vi "sub vi - calibration v1.vi"(11 "Temp Test Cal":dbl) -> ()   [LabVIEW 2013]
uses:
  <vilib>/Platform/TimedLoop/XDataNode/timing_clust.ctl
  <vilib>/Platform/TimedLoop/XDataNode/nitl_modes.ctl
  <vilib>/Platform/TimedLoop/XDataNode/wakeup.ctl
  <vilib>/platform/TimedLoop/XDataNode/XDataNode.xnode
  <vilib>/Platform/TimedLoop/XDataNode/XDNodeRunTimeDep.lvlib
panel:
  out "UPDATE":bool
  in  "stop":bool
  in  "Tab Control":T1(tab)
  out "1-2(TN) Run":dbl
  out "1-2(TL) Run":dbl
  out "1-1(TN) Run":dbl
  out "1-1(TL) Run":dbl
  out "LAB01-1 (GRAPH)":dynamicdata(graph)
  out "LAB01-2 (GRAPH)":dynamicdata(graph)
  in  "LAB01 (CAL)":T2 {"2 (TN) cal" min=0.0 step=0.01 format="%.2f"; "2 (TL) cal" min=0.0 step=0.01 format="%.2f"; "2 (PF) cal" min=0.0 step=0.01 format="%.2f"; "2 (V) cal" min=0.0 step=0.01 format="%.2f"; "2 (A) cal" min=0.0 step=0.01 format="%.2f"; "1 (TN) cal" min=0.0 step=0.01 format="%.2f"; "1 (TL) cal" min=0.0 step=0.01 format="%.2f"; "1 (PF) cal" min=0.0 step=0.01 format="%.2f"; "1 (V) cal" min=0.0 step=0.01 format="%.2f"; "1  (A) cal" min=0.0 step=0.01 format="%.2f"}
  out "LAB01 (SIGNALS)":T3 {"2 (PF)" format="%.2f"; "2 (A)" format="%.1f"; "1 (PF)" format="%.2f"; "1 (A)" format="%.1f"}
  out "2-2(TN) Run":dbl
  out "2-2(TL) Run":dbl
  out "2-1(TN) Run":dbl
  out "2-1(TL) Run":dbl
  out "LAB02 (SIGNALS)":T3 {"2 (PF)" format="%.2f"; "2 (A)" format="%.1f"; "1 (PF)" format="%.2f"; "1 (A)" format="%.1f"}
  in  "LAB02 (CAL)":T4 {"2 (TN) cal" min=0.0 step=0.01 format="%.2f"; "2 (TL) cal" min=0.0 step=0.01 format="%.2f"; "2 (PF) cal" min=0.0 step=0.01 format="%.2f"; "2 (V) cal" min=0.0 step=0.01 format="%.2f"; "2 (A) cal" min=0.0 step=0.01 format="%.2f"; "1 (TN) cal" min=0.0 step=0.01 format="%.2f"; "1 (TL) cal" min=0.0 step=0.01 format="%.2f"; "1 (PF) cal" min=0.0 step=0.01 format="%.2f"; "1 (V) cal" min=0.0 step=0.01 format="%.2f"; "1 (A) cal" min=0.0 step=0.01 format="%.2f"}
  out "LAB02-2 (GRAPH)":dynamicdata(graph)
  out "LAB02-1 (GRAPH)":dynamicdata(graph)
  out "3-2(TN) Run":dbl
  out "3-2(TL) Run":dbl
  out "3-1(TN) Run":dbl
  out "3-1(TL) Run":dbl
  out "LAB03 (SIGNALS)":T3 {"2 (PF)" format="%.2f"; "2 (A)" format="%.1f"; "1 (PF)" format="%.2f"; "1 (A)" format="%.1f"}
  in  "LAB03 (CAL)":T2 {"2 (TN) cal" min=0.0 step=0.01 format="%.2f"; "2 (TL) cal" min=0.0 step=0.01 format="%.2f"; "2 (PF) cal" min=0.0 step=0.01 format="%.2f"; "2 (V) cal" min=0.0 step=0.01 format="%.2f"; "2 (A) cal" min=0.0 step=0.01 format="%.2f"; "1 (TN) cal" min=0.0 step=0.01 format="%.2f"; "1 (TL) cal" min=0.0 step=0.01 format="%.2f"; "1 (PF) cal" min=0.0 step=0.01 format="%.2f"; "1 (V) cal" min=0.0 step=0.01 format="%.2f"; "1  (A) cal" min=0.0 step=0.01 format="%.2f"}
  out "LAB03-2 (GRAPH)":dynamicdata(graph)
  out "LAB03-1 (GRAPH)":dynamicdata(graph)
  out "4-2(TN) Run":dbl
  out "4-2(TL) Run":dbl
  out "4-1(TN) Run":dbl
  out "4-1(TL) Run":dbl
  out "LAB04 (SIGNALS)":T3 {"2 (PF)" format="%.2f"; "2 (A)" format="%.1f"; "1 (PF)" format="%.2f"; "1 (A)" format="%.1f"}
  in  "LAB04 (CAL)":T2 {"2 (TN) cal" min=0.0 step=0.01 format="%.2f"; "2 (TL) cal" min=0.0 step=0.01 format="%.2f"; "2 (PF) cal" min=0.0 step=0.01 format="%.2f"; "2 (V) cal" min=0.0 step=0.01 format="%.2f"; "2 (A) cal" min=0.0 step=0.01 format="%.2f"; "1 (TN) cal" min=0.0 step=0.01 format="%.2f"; "1 (TL) cal" min=0.0 step=0.01 format="%.2f"; "1 (PF) cal" min=0.0 step=0.01 format="%.2f"; "1 (V) cal" min=0.0 step=0.01 format="%.2f"; "1  (A) cal" min=0.0 step=0.01 format="%.2f"}
  out "LAB04-2 (GRAPH)":dynamicdata(graph)
  out "LAB04-1 (GRAPH)":dynamicdata(graph)
  out "5-2(TN) Run":dbl
  out "5-2(TL) Run":dbl
  out "5-1(TN) Run":dbl
  out "5-1(TL) Run":dbl
  out "LAB05 (SIGNALS)":T3 {"2 (PF)" format="%.2f"; "2 (A)" format="%.1f"; "1 (PF)" format="%.2f"; "1 (A)" format="%.1f"}
  in  "LAB05 (CAL)":T2 {"2 (TN) cal" min=0.0 step=0.01 format="%.2f"; "2 (TL) cal" min=0.0 step=0.01 format="%.2f"; "2 (PF) cal" min=0.0 step=0.01 format="%.2f"; "2 (V) cal" min=0.0 step=0.01 format="%.2f"; "2 (A) cal" min=0.0 step=0.01 format="%.2f"; "1 (TN) cal" min=0.0 step=0.01 format="%.2f"; "1 (TL) cal" min=0.0 step=0.01 format="%.2f"; "1 (PF) cal" min=0.0 step=0.01 format="%.2f"; "1 (V) cal" min=0.0 step=0.01 format="%.2f"; "1  (A) cal" min=0.0 step=0.01 format="%.2f"}
  out "LAB05-2 (GRAPH)":dynamicdata(graph)
  out "LAB05-1 (GRAPH)":dynamicdata(graph)
  in  "TEMP REF cal":dbl
  out "AMBIENT TEMP REF":dbl format="%.1f"
  out "Temperature data error":bool
  out "file error out":errorcluster
  out "Analog Loop Time":dbl
  out "analog read ERROR":errorcluster[](array[cluster])
  # "This value is only applied during\ntesting to adjust for insulatred probe\nprofile during current flow temp rise.\nIf any change is made here, make sure\nvalue is changed to same value on\nADM tab."
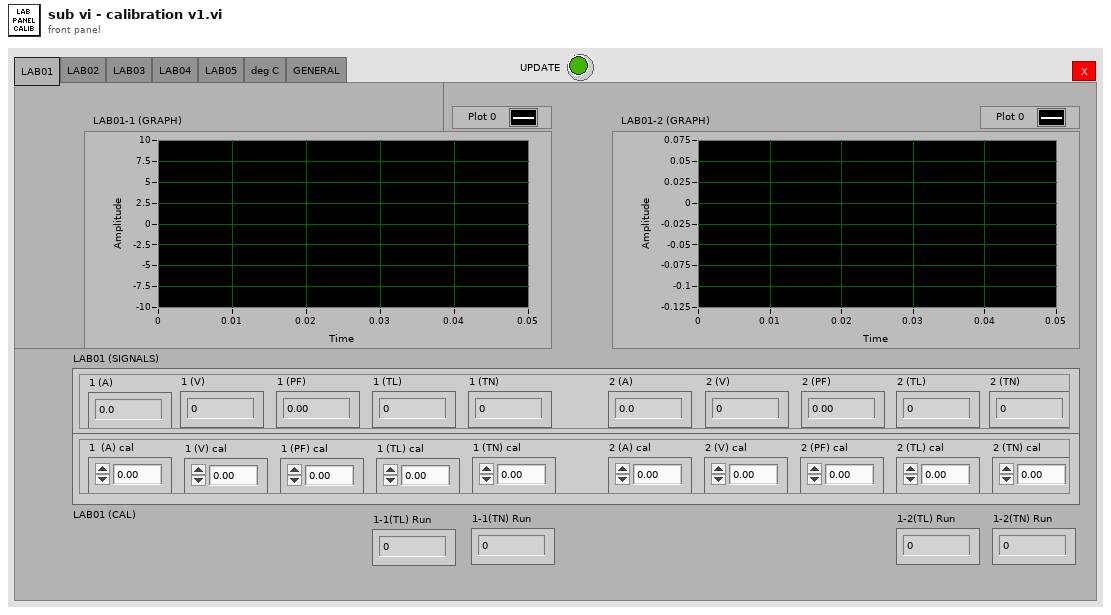
[diagram p1: front panel]
types:
  T1 = enum32{"LAB01", "LAB02", "LAB03", "LAB04", "LAB05", "deg C", "GENERAL"}
  T2 = cluster{"1  (A) cal":dbl, "1 (V) cal":dbl, "1 (PF) cal":dbl, "1 (TL) cal":dbl, "1 (TN) cal":dbl, "2 (A) cal":dbl, "2 (V) cal":dbl, "2 (PF) cal":dbl, "2 (TL) cal":dbl, "2 (TN) cal":dbl}
  T3 = cluster{"1 (TL)":dbl, "1 (TN)":dbl, "2 (TL)":dbl, "2 (TN)":dbl, "1 (A)":dbl, "1 (V)":dbl, "1 (PF)":dbl, "2 (A)":dbl, "2 (V)":dbl, "2 (PF)":dbl}
  T4 = cluster{"1 (A) cal":dbl, "1 (V) cal":dbl, "1 (PF) cal":dbl, "1 (TL) cal":dbl, "1 (TN) cal":dbl, "2 (A) cal":dbl, "2 (V) cal":dbl, "2 (PF) cal":dbl, "2 (TL) cal":dbl, "2 (TN) cal":dbl}
  T5 = enum16{"open", "replace", "create", "open or create", "replace or create", "replace or create with confirmation"}
  T6 = typedef "XDNodeRunTimeDep.lvlib/timing_clust.ctl" = cluster{"Expected End [f-1]":u64, "Actual End [f-1]":u64, "Finished Late? [f-1]":bool, "Expected End [i-1]":u64, "Actual End [i-1]":u64, "Finished Late? [i-1]":bool, "Expected Start [i]":u64, "Actual Start [i]":u64, "Expected Start [f]":u64, "Actual Start [f]":u64, "Source Name":string, "Structure Name":string, "Period":i64, "Deadline":i64, "Offset":i64, "Start":i64, "Priority":i32, "Timeout":i32, "Mode":T7, "Wakeup Reason":T8, "Error":errorcluster, "Source Type":string, "Secondary Source Type":string, "Global End Time":u64, "Global Start Time":u64, "Frame Duration":u64, "Iteration Duration":u64, "Assigned CPU":i32, "I/O Scan Engine Mode":u32}
  T7 = typedef "XDNodeRunTimeDep.lvlib/nitl_modes.ctl" = enum32{"No Change", "Process missed periods, maintain original phase", "Discard missed periods, maintain original phase", "Process missed periods, ignore original phase", "Discard missed periods, ignore original phase"}
  T8 = typedef "XDNodeRunTimeDep.lvlib/wakeup.ctl" = enum32{"Normal", "Aborted", "Asynchronous wakeup", "Timing source error", "Timed loop error", "Timeout"}
  T9 = cluster{"LAB01-1 (A)":dbl, "LAB01-1 (V)":dbl, "LAB01-1 (PF)":dbl, "LAB01-2 (A)":dbl, "LAB01-2 (V)":dbl, "LAB01-2 (PF)":dbl}
  T10 = cluster{"LAB02-1 (A)":dbl, "LAB02-1 (V)":dbl, "LAB02-1 (PF)":dbl, "LAB02-2 (A)":dbl, "LAB02-2 (V)":dbl, "LAB02-2 (PF)":dbl}
  T11 = cluster{"LAB03-1 (A)":dbl, "LAB03-1 (V)":dbl, "LAB03-1 (PF)":dbl, "LAB03-2 (A)":dbl, "LAB03-2 (V)":dbl, "LAB03-2 (PF)":dbl}
  T12 = cluster{"LAB04-1 (A)":dbl, "LAB04-1 (V)":dbl, "LAB04-1 (PF)":dbl, "LAB04-2 (A)":dbl, "LAB04-2 (V)":dbl, "LAB04-2 (PF)":dbl}
  T13 = cluster{"LAB05-1 (A)":dbl, "LAB05-1 (V)":dbl, "LAB05-1 (PF)":dbl, "LAB05-2 (A)":dbl, "LAB05-2 (V)":dbl, "LAB05-2 (PF)":dbl}
  T14 = cluster{"T1":dbl, "T2":dbl, "T3":dbl, "T4":dbl, "ID":dbl, "ER":dbl}
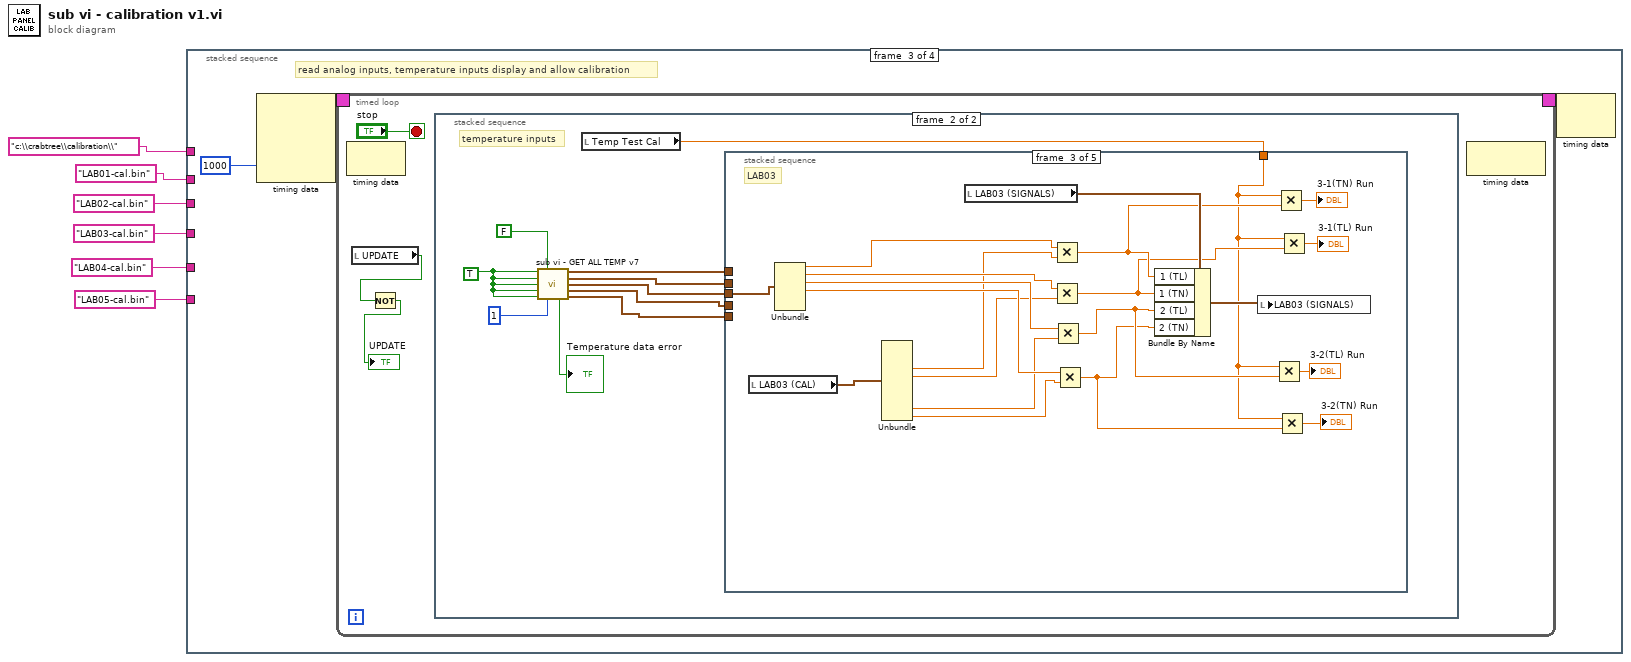
[diagram p0: block diagram]
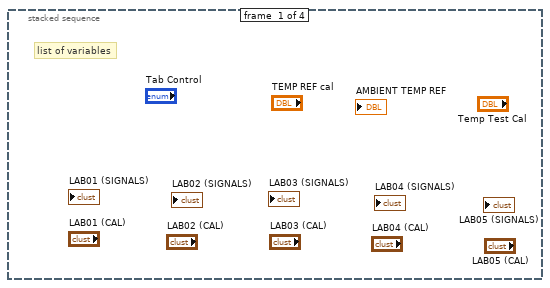
[diagram p2: hidden frame]
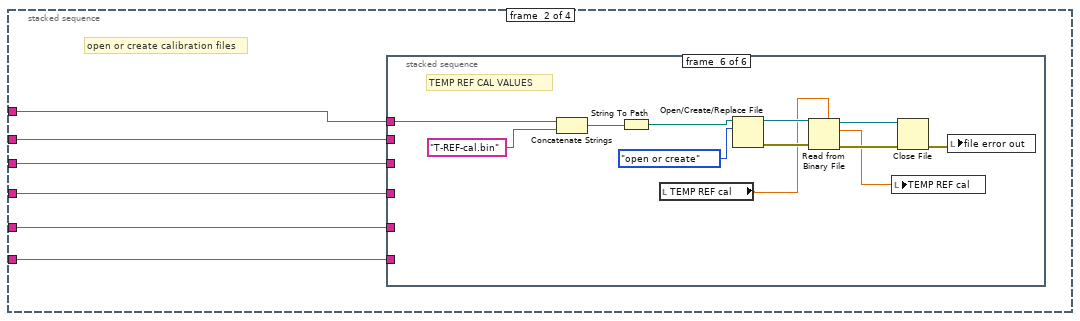
[diagram p3: hidden frame]
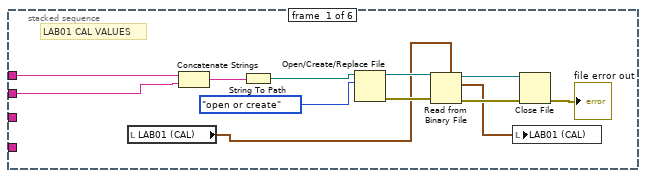
[diagram p4: hidden frame]
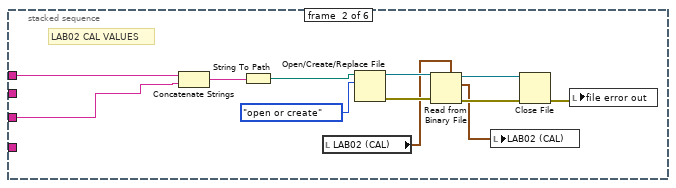
[diagram p5: hidden frame]
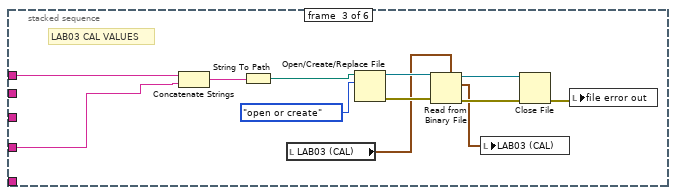
[diagram p6: hidden frame]
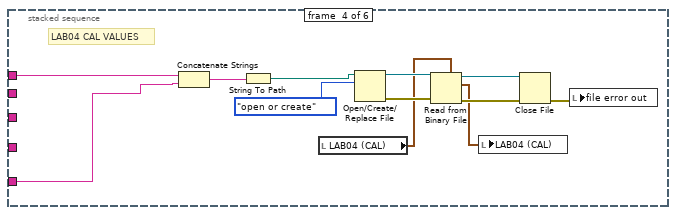
[diagram p7: hidden frame]
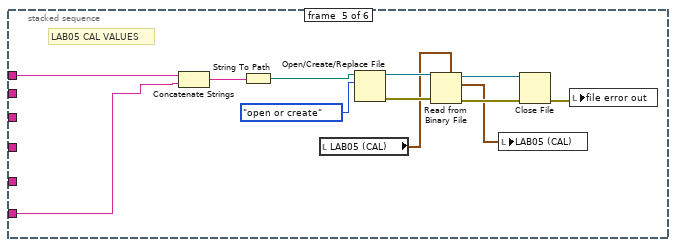
[diagram p8: hidden frame]
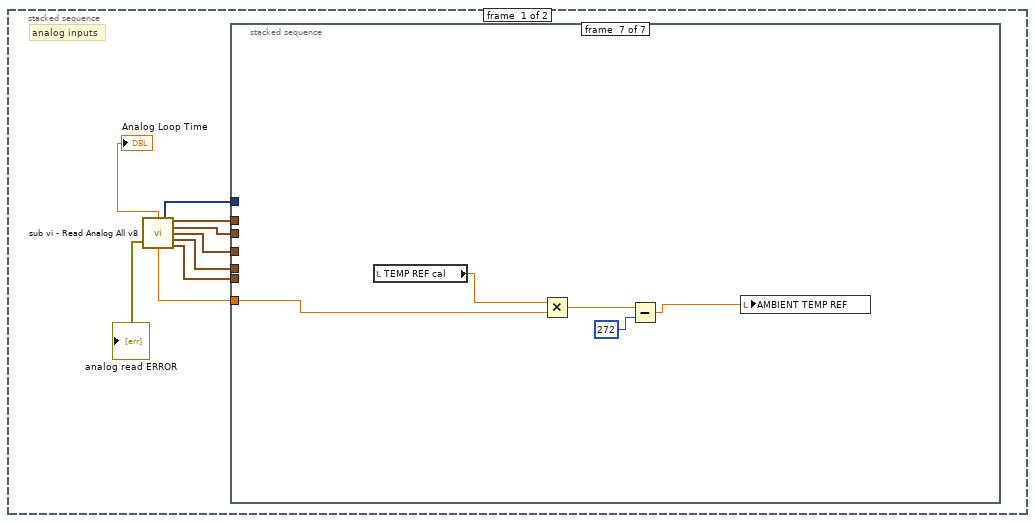
[diagram p9: hidden frame]
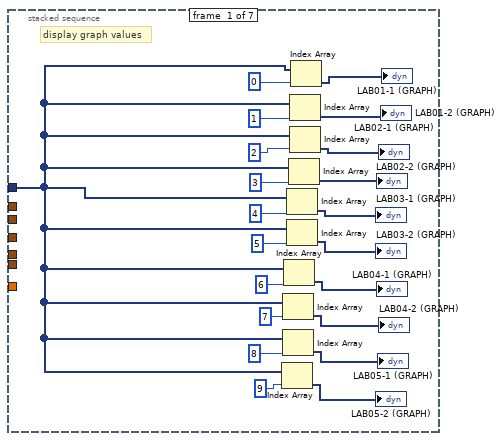
[diagram p10: hidden frame]
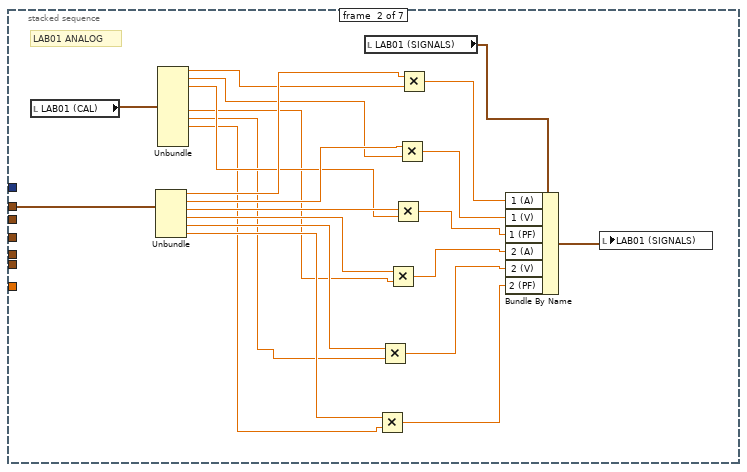
[diagram p11: hidden frame]
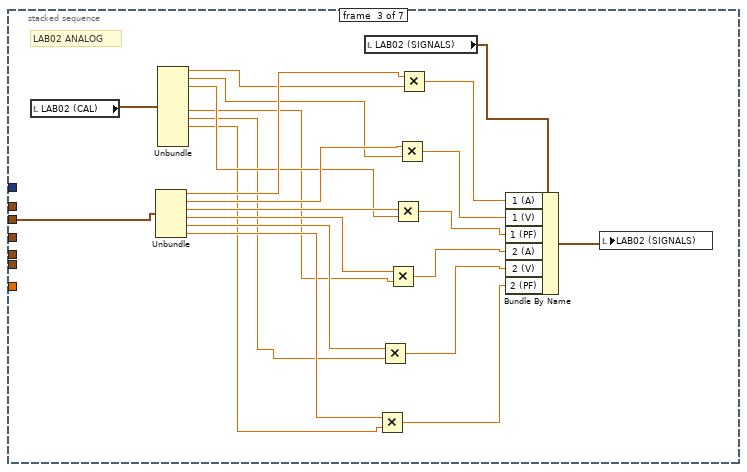
[diagram p12: hidden frame]
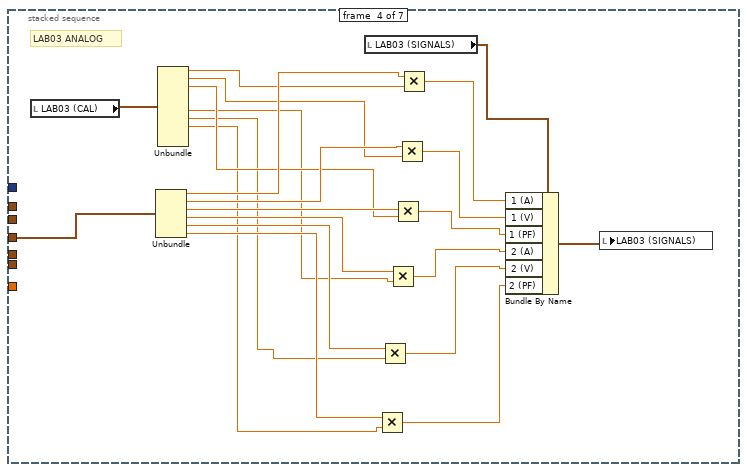
[diagram p13: hidden frame]
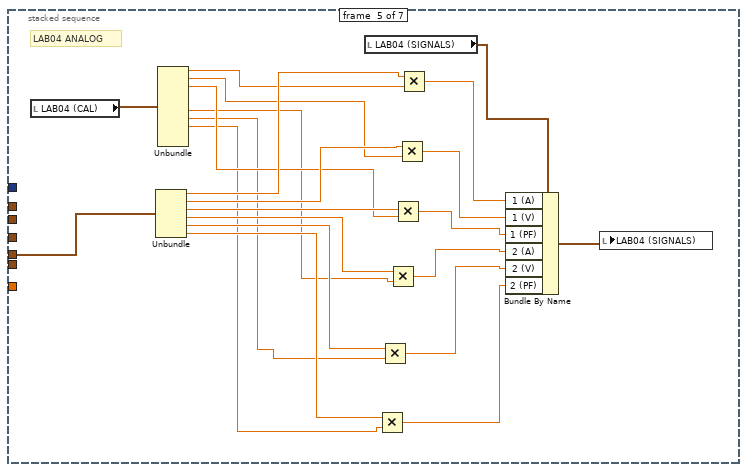
[diagram p14: hidden frame]
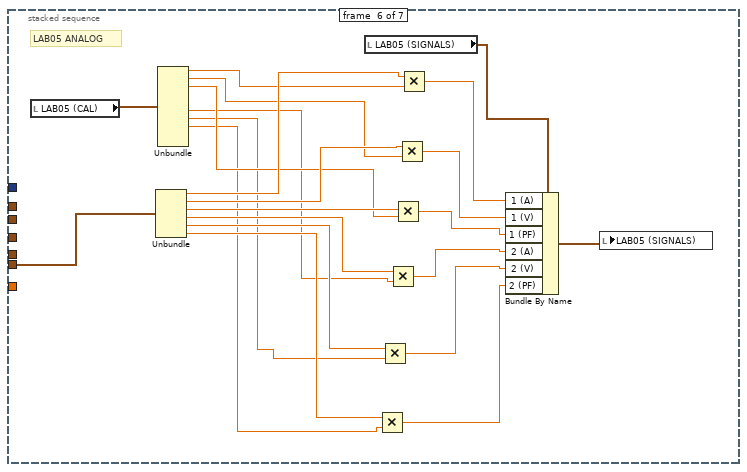
[diagram p15: hidden frame]
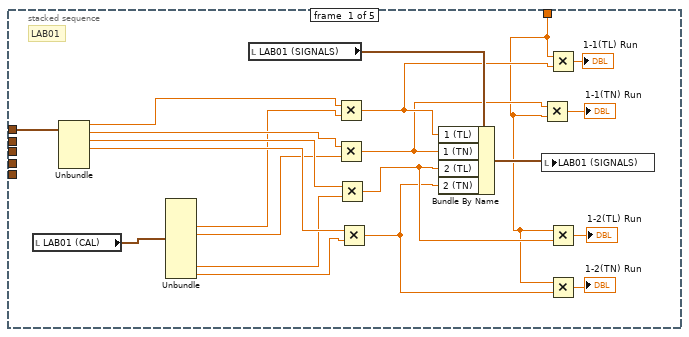
[diagram p16: hidden frame]
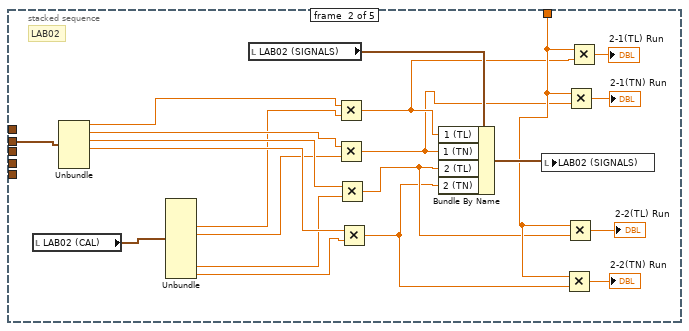
[diagram p17: hidden frame]
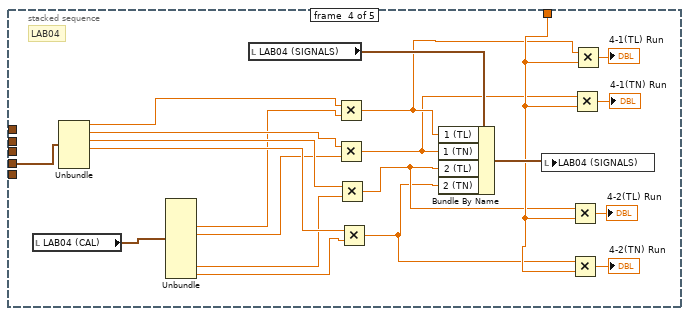
[diagram p18: hidden frame]
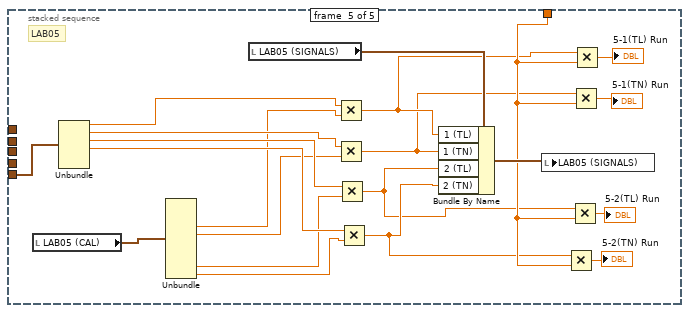
[diagram p19: hidden frame]
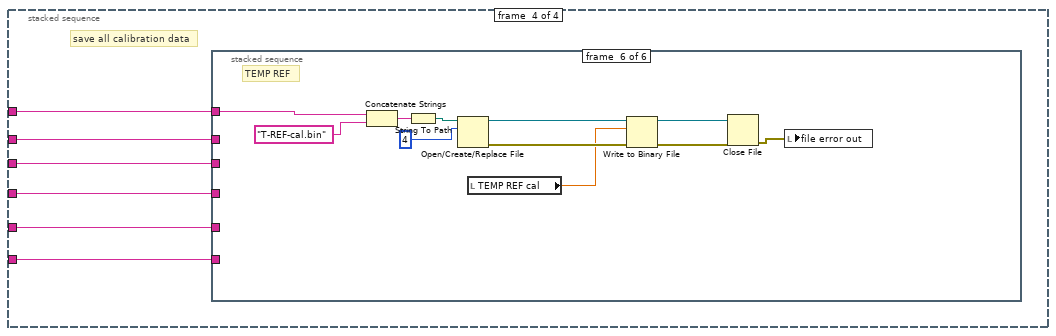
[diagram p20: hidden frame]
diagram:
  n1 = stacked-sequence {
    tunnel: "c:\\crabtree\\calibration\\" -> [_ w12 _ w362]
    tunnel: "LAB01-cal.bin" -> [_ w11 _ w361]
    tunnel: "LAB02-cal.bin" -> [_ w10 _ w360]
    tunnel: "LAB03-cal.bin" -> [_ w9 _ w359]
    tunnel: "LAB04-cal.bin" -> [_ w8 _ w358]
    tunnel: "LAB05-cal.bin" -> [_ w7 _ w357]
    frame #0 {
      # "list of variables"
    }
    frame #1 {
      # "open or create calibration files"
      n2 = stacked-sequence {
        tunnel: w12 -> [w24 w36 w48 w60 w72 w84]
        tunnel: w11 -> [w15 _ _ _ _ _]
        tunnel: w10 -> [_ w27 _ _ _ _]
        tunnel: w9 -> [_ _ w39 _ _ _]
        tunnel: w8 -> [_ _ _ w52 _ _]
        tunnel: w7 -> [_ _ _ _ w63 _]
        frame #0 {
          # "LAB01 CAL VALUES"
          n3 = local read "LAB01 (CAL)"() -> (w14:T2)
          n4 = Concatenate Strings(w24, w15) -> (w23:string)
          n5 = String To Path(string=w23) -> (path=w22:path)
          n6 = Open/Create/Replace File(file path (use dialog)=w22, operation (0:open)=T5."open or create") -> (refnum out=w21:refnum<file>, error out=w20:errorcluster)  [unwired: 4 in, 1 out]
          n7 = Read from Binary File(5:w14, 8:w20, 11:w21) -> (0:w18:errorcluster, 2:w13:T2, 3:w19:refnum<file>)  [unwired: 3 in, 1 out]
          n8 = local write "LAB01 (CAL)"(w13) -> ()
          n9 = Close File(refnum=w19, error in=w18) -> (error out=→"file error out":errorcluster)  [unwired: 1 out]
        }
        frame #1 {
          # "LAB02 CAL VALUES"
          n10 = Concatenate Strings(w36, w27) -> (w35:string)
          n11 = String To Path(string=w35) -> (path=w34:path)
          n12 = local read "LAB02 (CAL)"() -> (w26:T4)
          n13 = Open/Create/Replace File(file path (use dialog)=w34, operation (0:open)=T5."open or create") -> (refnum out=w33:refnum<file>, error out=w32:errorcluster)  [unwired: 4 in, 1 out]
          n14 = Read from Binary File(5:w26, 8:w32, 11:w33) -> (0:w30:errorcluster, 2:w25:T4, 3:w31:refnum<file>)  [unwired: 3 in, 1 out]
          n15 = local write "LAB02 (CAL)"(w25) -> ()
          n16 = Close File(refnum=w31, error in=w30) -> (error out=w28:errorcluster)  [unwired: 1 out]
          n17 = local write "file error out"(w28) -> ()
        }
        frame #2 {
          # "LAB03 CAL VALUES"
          n18 = Concatenate Strings(w48, w39) -> (w47:string)
          n19 = String To Path(string=w47) -> (path=w46:path)
          n20 = local read "LAB03 (CAL)"() -> (w38:T2)
          n21 = Open/Create/Replace File(file path (use dialog)=w46, operation (0:open)=T5."open or create") -> (refnum out=w45:refnum<file>, error out=w44:errorcluster)  [unwired: 4 in, 1 out]
          n22 = Read from Binary File(5:w38, 8:w44, 11:w45) -> (0:w42:errorcluster, 2:w37:T2, 3:w43:refnum<file>)  [unwired: 3 in, 1 out]
          n23 = local write "LAB03 (CAL)"(w37) -> ()
          n24 = Close File(refnum=w43, error in=w42) -> (error out=w40:errorcluster)  [unwired: 1 out]
          n25 = local write "file error out"(w40) -> ()
        }
        frame #3 {
          # "LAB04 CAL VALUES"
          n26 = Concatenate Strings(w60, w52) -> (w59:string)
          n27 = String To Path(string=w59) -> (path=w58:path)
          n28 = local read "LAB04 (CAL)"() -> (w50:T2)
          n29 = Open/Create/Replace File(file path (use dialog)=w58, operation (0:open)=T5."open or create") -> (refnum out=w57:refnum<file>, error out=w56:errorcluster)  [unwired: 4 in, 1 out]
          n30 = Read from Binary File(5:w50, 8:w56, 11:w57) -> (0:w54:errorcluster, 2:w49:T2, 3:w55:refnum<file>)  [unwired: 3 in, 1 out]
          n31 = local write "LAB04 (CAL)"(w49) -> ()
          n32 = Close File(refnum=w55, error in=w54) -> (error out=w53:errorcluster)  [unwired: 1 out]
          n33 = local write "file error out"(w53) -> ()
        }
        frame #4 {
          # "LAB05 CAL VALUES"
          n34 = Concatenate Strings(w72, w63) -> (w71:string)
          n35 = String To Path(string=w71) -> (path=w70:path)
          n36 = local read "LAB05 (CAL)"() -> (w62:T2)
          n37 = Open/Create/Replace File(file path (use dialog)=w70, operation (0:open)=T5."open or create") -> (refnum out=w69:refnum<file>, error out=w68:errorcluster)  [unwired: 4 in, 1 out]
          n38 = Read from Binary File(5:w62, 8:w68, 11:w69) -> (0:w66:errorcluster, 2:w61:T2, 3:w67:refnum<file>)  [unwired: 3 in, 1 out]
          n39 = local write "LAB05 (CAL)"(w61) -> ()
          n40 = Close File(refnum=w67, error in=w66) -> (error out=w64:errorcluster)  [unwired: 1 out]
          n41 = local write "file error out"(w64) -> ()
        }
        frame #5 {
          # "TEMP REF CAL VALUES"
          n42 = Concatenate Strings(w84, "T-REF-cal.bin") -> (w83:string)
          n43 = String To Path(string=w83) -> (path=w82:path)
          n44 = local read "TEMP REF cal"() -> (w74:dbl)
          n45 = Open/Create/Replace File(file path (use dialog)=w82, operation (0:open)=T5."open or create") -> (refnum out=w81:refnum<file>, error out=w80:errorcluster)  [unwired: 4 in, 1 out]
          n46 = Read from Binary File(5:w74, 8:w80, 11:w81) -> (0:w78:errorcluster, 2:w73:dbl, 3:w79:refnum<file>)  [unwired: 3 in, 1 out]
          n47 = local write "TEMP REF cal"(w73) -> ()
          n48 = Close File(refnum=w79, error in=w78) -> (error out=w76:errorcluster)  [unwired: 1 out]
          n49 = local write "file error out"(w76) -> ()
        }
      }
    }
    frame #2 {
      # "read analog inputs, temperature inputs display and allow calibration"
      n50 = node-c288(1000) -> (w87:T6)  [unwired: 3 in]
      n51 = timed-loop {
        timing: w87 -> [_]
        timing-out: [_] -> w86
        stop <- "stop" stop-if-true
        n52 = node-c288() -> ()  [unwired: 1 in, 1 out]
        n53 = local read "UPDATE"() -> (w88:bool)
        n54 = Not(x=w88) -> (.not. x?=→"UPDATE":bool)
        n55 = stacked-sequence {
          frame #0 {
            # "analog inputs"
            n56 = call "sub vi - Read Analog All v8.vi"() -> ("Analog loop time"=→"Analog Loop Time":dbl, "array GRAPH"=w98:dynamicdata[], "LAB01"=w97:T9, "LAB02"=w95:T10, "LAB03"=w96:T11, "LAB04"=w94:T12, "deg C"=w91:dbl, "array ERROR"=→"analog read ERROR":errorcluster[], "LAB05"=w93:T13)  [unwired: 7 in]
            n57 = stacked-sequence {
              tunnel: w98 -> [w119 _ _ _ _ _ _]
              tunnel: w97 -> [_ w141 _ _ _ _ _]
              tunnel: w96 -> [_ _ _ w165 _ _ _]
              tunnel: w95 -> [_ _ w143 _ _ _ _]
              tunnel: w94 -> [_ _ _ _ w187 _ _]
              tunnel: w93 -> [_ _ _ _ _ w209 _]
              tunnel: w91 -> [_ _ _ _ _ _ w234]
              frame #0 {
                # "display graph values"
                n58 = Index Array(array=w119, index=9) -> (element=→"LAB05-2 (GRAPH)":dynamicdata)
                n59 = Index Array(array=w119, index=7) -> (element=→"LAB04-2 (GRAPH)":dynamicdata)
                n60 = Index Array(array=w119, index=8) -> (element=→"LAB05-1 (GRAPH)":dynamicdata)
                n61 = Index Array(array=w119, index=6) -> (element=→"LAB04-1 (GRAPH)":dynamicdata)
                n62 = Index Array(array=w119, index=4) -> (element=→"LAB03-1 (GRAPH)":dynamicdata)
                n63 = Index Array(array=w119, index=5) -> (element=→"LAB03-2 (GRAPH)":dynamicdata)
                n64 = Index Array(array=w119, index=3) -> (element=→"LAB02-2 (GRAPH)":dynamicdata)
                n65 = Index Array(array=w119, index=1) -> (element=→"LAB01-2 (GRAPH)":dynamicdata)
                n66 = Index Array(array=w119, index=2) -> (element=→"LAB02-1 (GRAPH)":dynamicdata)
                n67 = Index Array(array=w119, index=0) -> (element=→"LAB01-1 (GRAPH)":dynamicdata)
              }
              frame #1 {
                # "LAB01 ANALOG"
                n68 = local read "LAB01 (CAL)"() -> (w142:T2)
                n69 = Unbundle(w141) -> ("LAB01-1 (A)"=w140:dbl, "LAB01-1 (V)"=w139:dbl, "LAB01-1 (PF)"=w138:dbl, "LAB01-2 (A)"=w137:dbl, "LAB01-2 (V)"=w136:dbl, "LAB01-2 (PF)"=w135:dbl)
                n70 = Unbundle(w142) -> ("1  (A) cal"=w134:dbl, "1 (V) cal"=w133:dbl, "1 (PF) cal"=w132:dbl, "2 (A) cal"=w131:dbl, "2 (V) cal"=w130:dbl, "2 (PF) cal"=w129:dbl)  [unwired: 4 out]
                n71 = local read "LAB01 (SIGNALS)"() -> (w128:T3)
                n72 = Multiply(x=w135, y=w129) -> (x*y=w122:dbl)
                n73 = Multiply(x=w136, y=w130) -> (x*y=w123:dbl)
                n74 = Multiply(x=w137, y=w131) -> (x*y=w124:dbl)
                n75 = Multiply(x=w138, y=w132) -> (x*y=w125:dbl)
                n76 = Multiply(x=w139, y=w133) -> (x*y=w126:dbl)
                n77 = Multiply(x=w140, y=w134) -> (x*y=w127:dbl)
                n78 = Bundle By Name(cluster=w128, "1 (A)"=w127, "1 (V)"=w126, "1 (PF)"=w125, "2 (A)"=w124, "2 (V)"=w123, "2 (PF)"=w122) -> (w121:T3)
                n79 = local write "LAB01 (SIGNALS)"(w121) -> ()
              }
              frame #2 {
                # "LAB02 ANALOG"
                n80 = local read "LAB02 (CAL)"() -> (w164:T4)
                n81 = Unbundle(w143) -> ("LAB02-1 (A)"=w163:dbl, "LAB02-1 (V)"=w162:dbl, "LAB02-1 (PF)"=w161:dbl, "LAB02-2 (A)"=w160:dbl, "LAB02-2 (V)"=w159:dbl, "LAB02-2 (PF)"=w158:dbl)
                n82 = Unbundle(w164) -> ("1 (A) cal"=w157:dbl, "1 (V) cal"=w156:dbl, "1 (PF) cal"=w155:dbl, "2 (A) cal"=w154:dbl, "2 (V) cal"=w153:dbl, "2 (PF) cal"=w152:dbl)  [unwired: 4 out]
                n83 = local read "LAB02 (SIGNALS)"() -> (w151:T3)
                n84 = Multiply(x=w158, y=w152) -> (x*y=w145:dbl)
                n85 = Multiply(x=w159, y=w153) -> (x*y=w146:dbl)
                n86 = Multiply(x=w160, y=w154) -> (x*y=w147:dbl)
                n87 = Multiply(x=w161, y=w155) -> (x*y=w148:dbl)
                n88 = Multiply(x=w162, y=w156) -> (x*y=w149:dbl)
                n89 = Multiply(x=w163, y=w157) -> (x*y=w150:dbl)
                n90 = Bundle By Name(cluster=w151, "1 (A)"=w150, "1 (V)"=w149, "1 (PF)"=w148, "2 (A)"=w147, "2 (V)"=w146, "2 (PF)"=w145) -> (w144:T3)
                n91 = local write "LAB02 (SIGNALS)"(w144) -> ()
              }
              frame #3 {
                # "LAB03 ANALOG"
                n92 = local read "LAB03 (CAL)"() -> (w186:T2)
                n93 = Unbundle(w165) -> ("LAB03-1 (A)"=w185:dbl, "LAB03-1 (V)"=w184:dbl, "LAB03-1 (PF)"=w183:dbl, "LAB03-2 (A)"=w182:dbl, "LAB03-2 (V)"=w181:dbl, "LAB03-2 (PF)"=w180:dbl)
                n94 = Unbundle(w186) -> ("1  (A) cal"=w179:dbl, "1 (V) cal"=w178:dbl, "1 (PF) cal"=w177:dbl, "2 (A) cal"=w176:dbl, "2 (V) cal"=w175:dbl, "2 (PF) cal"=w174:dbl)  [unwired: 4 out]
                n95 = local read "LAB03 (SIGNALS)"() -> (w173:T3)
                n96 = Multiply(x=w180, y=w174) -> (x*y=w167:dbl)
                n97 = Multiply(x=w181, y=w175) -> (x*y=w168:dbl)
                n98 = Multiply(x=w182, y=w176) -> (x*y=w169:dbl)
                n99 = Multiply(x=w183, y=w177) -> (x*y=w170:dbl)
                n100 = Multiply(x=w184, y=w178) -> (x*y=w171:dbl)
                n101 = Multiply(x=w185, y=w179) -> (x*y=w172:dbl)
                n102 = Bundle By Name(cluster=w173, "1 (A)"=w172, "1 (V)"=w171, "1 (PF)"=w170, "2 (A)"=w169, "2 (V)"=w168, "2 (PF)"=w167) -> (w166:T3)
                n103 = local write "LAB03 (SIGNALS)"(w166) -> ()
              }
              frame #4 {
                # "LAB04 ANALOG"
                n104 = local read "LAB04 (CAL)"() -> (w208:T2)
                n105 = Unbundle(w187) -> ("LAB04-1 (A)"=w207:dbl, "LAB04-1 (V)"=w206:dbl, "LAB04-1 (PF)"=w205:dbl, "LAB04-2 (A)"=w204:dbl, "LAB04-2 (V)"=w203:dbl, "LAB04-2 (PF)"=w202:dbl)
                n106 = Unbundle(w208) -> ("1  (A) cal"=w201:dbl, "1 (V) cal"=w200:dbl, "1 (PF) cal"=w199:dbl, "2 (A) cal"=w198:dbl, "2 (V) cal"=w197:dbl, "2 (PF) cal"=w196:dbl)  [unwired: 4 out]
                n107 = local read "LAB04 (SIGNALS)"() -> (w195:T3)
                n108 = Multiply(x=w202, y=w196) -> (x*y=w189:dbl)
                n109 = Multiply(x=w203, y=w197) -> (x*y=w190:dbl)
                n110 = Multiply(x=w204, y=w198) -> (x*y=w191:dbl)
                n111 = Multiply(x=w205, y=w199) -> (x*y=w192:dbl)
                n112 = Multiply(x=w206, y=w200) -> (x*y=w193:dbl)
                n113 = Multiply(x=w207, y=w201) -> (x*y=w194:dbl)
                n114 = Bundle By Name(cluster=w195, "1 (A)"=w194, "1 (V)"=w193, "1 (PF)"=w192, "2 (A)"=w191, "2 (V)"=w190, "2 (PF)"=w189) -> (w188:T3)
                n115 = local write "LAB04 (SIGNALS)"(w188) -> ()
              }
              frame #5 {
                # "LAB05 ANALOG"
                n116 = local read "LAB05 (CAL)"() -> (w230:T2)
                n117 = Unbundle(w209) -> ("LAB05-1 (A)"=w229:dbl, "LAB05-1 (V)"=w228:dbl, "LAB05-1 (PF)"=w227:dbl, "LAB05-2 (A)"=w226:dbl, "LAB05-2 (V)"=w225:dbl, "LAB05-2 (PF)"=w224:dbl)
                n118 = Unbundle(w230) -> ("1  (A) cal"=w223:dbl, "1 (V) cal"=w222:dbl, "1 (PF) cal"=w221:dbl, "2 (A) cal"=w220:dbl, "2 (V) cal"=w219:dbl, "2 (PF) cal"=w218:dbl)  [unwired: 4 out]
                n119 = local read "LAB05 (SIGNALS)"() -> (w217:T3)
                n120 = Multiply(x=w224, y=w218) -> (x*y=w211:dbl)
                n121 = Multiply(x=w225, y=w219) -> (x*y=w212:dbl)
                n122 = Multiply(x=w226, y=w220) -> (x*y=w213:dbl)
                n123 = Multiply(x=w227, y=w221) -> (x*y=w214:dbl)
                n124 = Multiply(x=w228, y=w222) -> (x*y=w215:dbl)
                n125 = Multiply(x=w229, y=w223) -> (x*y=w216:dbl)
                n126 = Bundle By Name(cluster=w217, "1 (A)"=w216, "1 (V)"=w215, "1 (PF)"=w214, "2 (A)"=w213, "2 (V)"=w212, "2 (PF)"=w211) -> (w210:T3)
                n127 = local write "LAB05 (SIGNALS)"(w210) -> ()
              }
              frame #6 {
                n128 = local read "TEMP REF cal"() -> (w235:dbl)
                n129 = Multiply(x=w235, y=w234) -> (x*y=w233:dbl)
                n130 = Subtract(x=w233, y=272) -> (x-y=w231:dbl)
                n131 = local write "AMBIENT TEMP REF"(w231) -> ()
              }
            }
          }
          frame #1 {
            w245 = TRUE
            # "temperature inputs"
            n132 = call "sub vi - GET ALL TEMP v7.vi"("LA01-EN"=w245, "simulate"=FALSE, "LA02-EN"=w245, "LA03-EN"=w245, "LA04-EN"=w245, "LA05-EN"=w245, "Gen Cal Value"=1) -> ("LA01 TEMP"=w243:T14, "LA02 TEMP"=w241:T14, "LA03 TEMP"=w240:T14, "LA04 TEMP"=w239:T14, "error"=→"Temperature data error":bool, "LA05 TEMP"=w238:T14)  [unwired: 1 in, 2 out]
            n133 = local read "Temp Test Cal"() -> (w236:dbl)
            n134 = stacked-sequence {
              tunnel: w243 -> [w265 _ _ _ _]
              tunnel: w241 -> [_ w276 _ _ _]
              tunnel: w240 -> [_ _ w297 _ _]
              tunnel: w239 -> [_ _ _ w318 _]
              tunnel: w238 -> [_ _ _ _ w339]
              tunnel: w236 -> [w246 w271 w289 w313 w334]
              frame #0 {
                # "LAB01"
                n135 = local read "LAB01 (CAL)"() -> (w266:T2)
                n136 = Unbundle(w265) -> ("T1"=w264:dbl, "T2"=w263:dbl, "T3"=w262:dbl, "T4"=w261:dbl)  [unwired: 2 out]
                n137 = Unbundle(w266) -> ("1 (TL) cal"=w260:dbl, "1 (TN) cal"=w259:dbl, "2 (TL) cal"=w258:dbl, "2 (TN) cal"=w257:dbl)  [unwired: 6 out]
                n138 = local read "LAB01 (SIGNALS)"() -> (w256:T3)
                n139 = Multiply(x=w264, y=w260) -> (x*y=w253:dbl)
                n140 = Multiply(x=w263, y=w259) -> (x*y=w251:dbl)
                n141 = Multiply(x=w262, y=w258) -> (x*y=w248:dbl)
                n142 = Multiply(x=w261, y=w257) -> (x*y=w247:dbl)
                n143 = Bundle By Name(cluster=w256, "1 (TL)"=w253, "1 (TN)"=w251, "2 (TL)"=w248, "2 (TN)"=w247) -> (w255:T3)
                n144 = Multiply(x=w251, y=w246) -> (x*y=→"1-1(TN) Run":dbl)
                n145 = local write "LAB01 (SIGNALS)"(w255) -> ()
                n146 = Multiply(x=w246, y=w253) -> (x*y=→"1-1(TL) Run":dbl)
                n147 = Multiply(x=w246, y=w248) -> (x*y=→"1-2(TL) Run":dbl)
                n148 = Multiply(x=w246, y=w247) -> (x*y=→"1-2(TN) Run":dbl)
              }
              frame #1 {
                # "LAB02"
                n149 = local read "LAB02 (CAL)"() -> (w287:T4)
                n150 = Unbundle(w276) -> ("T1"=w286:dbl, "T2"=w285:dbl, "T3"=w284:dbl, "T4"=w283:dbl)  [unwired: 2 out]
                n151 = Unbundle(w287) -> ("1 (TL) cal"=w282:dbl, "1 (TN) cal"=w281:dbl, "2 (TL) cal"=w280:dbl, "2 (TN) cal"=w279:dbl)  [unwired: 6 out]
                n152 = local read "LAB02 (SIGNALS)"() -> (w278:T3)
                n153 = Multiply(x=w286, y=w282) -> (x*y=w270:dbl)
                n154 = Multiply(x=w285, y=w281) -> (x*y=w269:dbl)
                n155 = Multiply(x=w284, y=w280) -> (x*y=w268:dbl)
                n156 = Multiply(x=w283, y=w279) -> (x*y=w267:dbl)
                n157 = Bundle By Name(cluster=w278, "1 (TL)"=w270, "1 (TN)"=w269, "2 (TL)"=w268, "2 (TN)"=w267) -> (w277:T3)
                n158 = local write "LAB02 (SIGNALS)"(w277) -> ()
                n159 = Multiply(x=w271, y=w267) -> (x*y=→"2-2(TN) Run":dbl)
                n160 = Multiply(x=w271, y=w268) -> (x*y=→"2-2(TL) Run":dbl)
                n161 = Multiply(x=w271, y=w269) -> (x*y=→"2-1(TN) Run":dbl)
                n162 = Multiply(x=w271, y=w270) -> (x*y=→"2-1(TL) Run":dbl)
              }
              frame #2 {
                # "LAB03"
                n163 = local read "LAB03 (CAL)"() -> (w308:T2)
                n164 = Unbundle(w297) -> ("T1"=w307:dbl, "T2"=w306:dbl, "T3"=w305:dbl, "T4"=w304:dbl)  [unwired: 2 out]
                n165 = Unbundle(w308) -> ("1 (TL) cal"=w303:dbl, "1 (TN) cal"=w302:dbl, "2 (TL) cal"=w301:dbl, "2 (TN) cal"=w300:dbl)  [unwired: 6 out]
                n166 = local read "LAB03 (SIGNALS)"() -> (w299:T3)
                n167 = Multiply(x=w307, y=w303) -> (x*y=w293:dbl)
                n168 = Multiply(x=w306, y=w302) -> (x*y=w292:dbl)
                n169 = Multiply(x=w305, y=w301) -> (x*y=w291:dbl)
                n170 = Multiply(x=w304, y=w300) -> (x*y=w290:dbl)
                n171 = Bundle By Name(cluster=w299, "1 (TL)"=w293, "1 (TN)"=w292, "2 (TL)"=w291, "2 (TN)"=w290) -> (w298:T3)
                n172 = local write "LAB03 (SIGNALS)"(w298) -> ()
                n173 = Multiply(x=w289, y=w291) -> (x*y=→"3-2(TL) Run":dbl)
                n174 = Multiply(x=w289, y=w293) -> (x*y=→"3-1(TN) Run":dbl)
                n175 = Multiply(x=w289, y=w290) -> (x*y=→"3-2(TN) Run":dbl)
                n176 = Multiply(x=w289, y=w292) -> (x*y=→"3-1(TL) Run":dbl)
              }
              frame #3 {
                # "LAB04"
                n177 = local read "LAB04 (CAL)"() -> (w329:T2)
                n178 = Unbundle(w318) -> ("T1"=w328:dbl, "T2"=w327:dbl, "T3"=w326:dbl, "T4"=w325:dbl)  [unwired: 2 out]
                n179 = Unbundle(w329) -> ("1 (TL) cal"=w324:dbl, "1 (TN) cal"=w323:dbl, "2 (TL) cal"=w322:dbl, "2 (TN) cal"=w321:dbl)  [unwired: 6 out]
                n180 = local read "LAB04 (SIGNALS)"() -> (w320:T3)
                n181 = Multiply(x=w328, y=w324) -> (x*y=w312:dbl)
                n182 = Multiply(x=w327, y=w323) -> (x*y=w311:dbl)
                n183 = Multiply(x=w326, y=w322) -> (x*y=w310:dbl)
                n184 = Multiply(x=w325, y=w321) -> (x*y=w309:dbl)
                n185 = Bundle By Name(cluster=w320, "1 (TL)"=w312, "1 (TN)"=w311, "2 (TL)"=w310, "2 (TN)"=w309) -> (w319:T3)
                n186 = local write "LAB04 (SIGNALS)"(w319) -> ()
                n187 = Multiply(x=w310, y=w313) -> (x*y=→"4-2(TL) Run":dbl)
                n188 = Multiply(x=w309, y=w313) -> (x*y=→"4-2(TN) Run":dbl)
                n189 = Multiply(x=w311, y=w313) -> (x*y=→"4-1(TN) Run":dbl)
                n190 = Multiply(x=w312, y=w313) -> (x*y=→"4-1(TL) Run":dbl)
              }
              frame #4 {
                # "LAB05"
                n191 = local read "LAB05 (CAL)"() -> (w350:T2)
                n192 = Unbundle(w339) -> ("T1"=w349:dbl, "T2"=w348:dbl, "T3"=w347:dbl, "T4"=w346:dbl)  [unwired: 2 out]
                n193 = Unbundle(w350) -> ("1 (TL) cal"=w345:dbl, "1 (TN) cal"=w344:dbl, "2 (TL) cal"=w343:dbl, "2 (TN) cal"=w342:dbl)  [unwired: 6 out]
                n194 = local read "LAB05 (SIGNALS)"() -> (w341:T3)
                n195 = Multiply(x=w349, y=w345) -> (x*y=w333:dbl)
                n196 = Multiply(x=w348, y=w344) -> (x*y=w332:dbl)
                n197 = Multiply(x=w347, y=w343) -> (x*y=w330:dbl)
                n198 = Multiply(x=w346, y=w342) -> (x*y=w331:dbl)
                n199 = Bundle By Name(cluster=w341, "1 (TL)"=w333, "1 (TN)"=w332, "2 (TL)"=w330, "2 (TN)"=w331) -> (w340:T3)
                n200 = local write "LAB05 (SIGNALS)"(w340) -> ()
                n201 = Multiply(x=w331, y=w334) -> (x*y=→"5-2(TN) Run":dbl)
                n202 = Multiply(x=w330, y=w334) -> (x*y=→"5-2(TL) Run":dbl)
                n203 = Multiply(x=w332, y=w334) -> (x*y=→"5-1(TN) Run":dbl)
                n204 = Multiply(x=w333, y=w334) -> (x*y=→"5-1(TL) Run":dbl)
              }
            }
          }
        }
        n205 = node-c288() -> ()  [unwired: 1 in, 1 out]
      }
      n206 = node-c288(w86) -> ()  [unwired: 1 out]
    }
    frame #3 {
      # "save all calibration data"
      n207 = stacked-sequence {
        tunnel: w362 -> [w372 w383 w394 w405 w416 w427]
        tunnel: w361 -> [w371 _ _ _ _ _]
        tunnel: w360 -> [_ w374 _ _ _ _]
        tunnel: w359 -> [_ _ w385 _ _ _]
        tunnel: w358 -> [_ _ _ w396 _ _]
        tunnel: w357 -> [_ _ _ _ w407 _]
        frame #0 {
          # "LAB01"
          n208 = Concatenate Strings(w372, w371) -> (w373:string)
          n209 = String To Path(string=w373) -> (path=w370:path)
          n210 = Open/Create/Replace File(file path (use dialog)=w370, operation (0:open)=4) -> (refnum out=w369:refnum<file>, error out=w368:errorcluster)  [unwired: 4 in, 1 out]
          n211 = local read "LAB01 (CAL)"() -> (w363:T2)
          n212 = Write to Binary File(file (use dialog)=w369, data=w363, error in=w368) -> (refnum out=w367:refnum<file>, error out=w366:errorcluster)  [unwired: 3 in, 1 out]
          n213 = Close File(refnum=w367, error in=w366) -> (error out=w365:errorcluster)  [unwired: 1 out]
          n214 = local write "file error out"(w365) -> ()
        }
        frame #1 {
          # "LAB02"
          n215 = Concatenate Strings(w383, w374) -> (w384:string)
          n216 = String To Path(string=w384) -> (path=w382:path)
          n217 = Open/Create/Replace File(file path (use dialog)=w382, operation (0:open)=4) -> (refnum out=w381:refnum<file>, error out=w380:errorcluster)  [unwired: 4 in, 1 out]
          n218 = local read "LAB02 (CAL)"() -> (w375:T4)
          n219 = Write to Binary File(file (use dialog)=w381, data=w375, error in=w380) -> (refnum out=w379:refnum<file>, error out=w378:errorcluster)  [unwired: 3 in, 1 out]
          n220 = Close File(refnum=w379, error in=w378) -> (error out=w377:errorcluster)  [unwired: 1 out]
          n221 = local write "file error out"(w377) -> ()
        }
        frame #2 {
          # "LAB03"
          n222 = Concatenate Strings(w394, w385) -> (w395:string)
          n223 = String To Path(string=w395) -> (path=w393:path)
          n224 = Open/Create/Replace File(file path (use dialog)=w393, operation (0:open)=4) -> (refnum out=w392:refnum<file>, error out=w391:errorcluster)  [unwired: 4 in, 1 out]
          n225 = local read "LAB03 (CAL)"() -> (w386:T2)
          n226 = Write to Binary File(file (use dialog)=w392, data=w386, error in=w391) -> (refnum out=w390:refnum<file>, error out=w389:errorcluster)  [unwired: 3 in, 1 out]
          n227 = Close File(refnum=w390, error in=w389) -> (error out=w388:errorcluster)  [unwired: 1 out]
          n228 = local write "file error out"(w388) -> ()
        }
        frame #3 {
          # "LAB04"
          n229 = Concatenate Strings(w405, w396) -> (w406:string)
          n230 = String To Path(string=w406) -> (path=w404:path)
          n231 = Open/Create/Replace File(file path (use dialog)=w404, operation (0:open)=4) -> (refnum out=w403:refnum<file>, error out=w402:errorcluster)  [unwired: 4 in, 1 out]
          n232 = local read "LAB04 (CAL)"() -> (w397:T2)
          n233 = Write to Binary File(file (use dialog)=w403, data=w397, error in=w402) -> (refnum out=w401:refnum<file>, error out=w400:errorcluster)  [unwired: 3 in, 1 out]
          n234 = Close File(refnum=w401, error in=w400) -> (error out=w399:errorcluster)  [unwired: 1 out]
          n235 = local write "file error out"(w399) -> ()
        }
        frame #4 {
          # "LAB05"
          n236 = Concatenate Strings(w416, w407) -> (w417:string)
          n237 = String To Path(string=w417) -> (path=w415:path)
          n238 = Open/Create/Replace File(file path (use dialog)=w415, operation (0:open)=4) -> (refnum out=w414:refnum<file>, error out=w413:errorcluster)  [unwired: 4 in, 1 out]
          n239 = local read "LAB05 (CAL)"() -> (w408:T2)
          n240 = Write to Binary File(file (use dialog)=w414, data=w408, error in=w413) -> (refnum out=w412:refnum<file>, error out=w411:errorcluster)  [unwired: 3 in, 1 out]
          n241 = Close File(refnum=w412, error in=w411) -> (error out=w410:errorcluster)  [unwired: 1 out]
          n242 = local write "file error out"(w410) -> ()
        }
        frame #5 {
          # "TEMP REF"
          n243 = Concatenate Strings(w427, "T-REF-cal.bin") -> (w428:string)
          n244 = String To Path(string=w428) -> (path=w426:path)
          n245 = Open/Create/Replace File(file path (use dialog)=w426, operation (0:open)=4) -> (refnum out=w425:refnum<file>, error out=w424:errorcluster)  [unwired: 4 in, 1 out]
          n246 = local read "TEMP REF cal"() -> (w419:dbl)
          n247 = Write to Binary File(file (use dialog)=w425, data=w419, error in=w424) -> (refnum out=w423:refnum<file>, error out=w422:errorcluster)  [unwired: 3 in, 1 out]
          n248 = Close File(refnum=w423, error in=w422) -> (error out=w421:errorcluster)  [unwired: 1 out]
          n249 = local write "file error out"(w421) -> ()
        }
      }
    }
  }
